vi "Exercise 2.2 DS18b20.vi"() -> ()   [LabVIEW 2014]
panel:
  out "Delay ms":u32
  out "C Chart":dbl(graph)=34.187
  out "C Meter":dbl(knob)=34.187 scale=15.0..40.0
  in  "error in (no error)":errorcluster
  out "error out":errorcluster
  out "Active":bool
  out "c":dbl=34.187
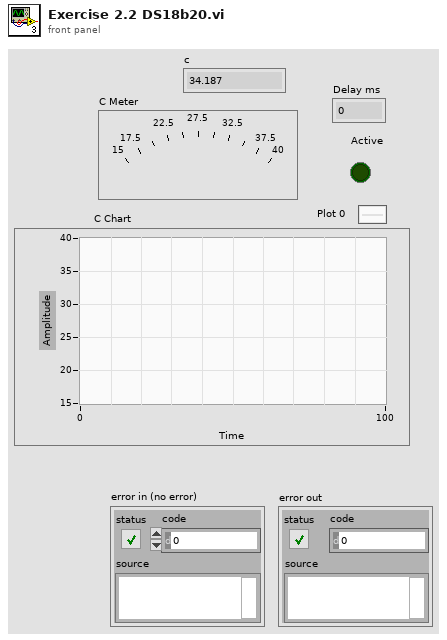
[diagram p1: front panel]
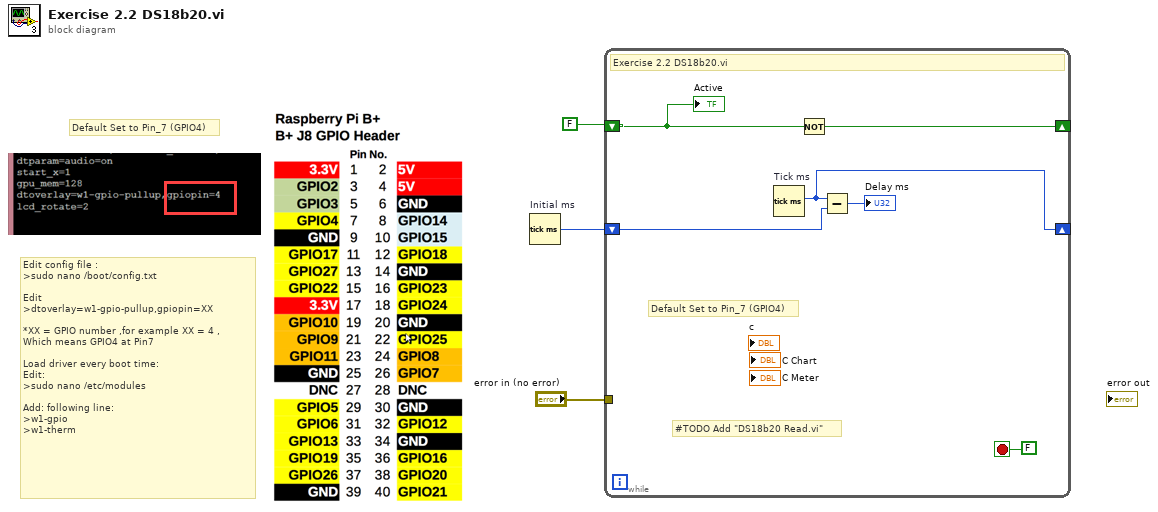
[diagram p0: block diagram]
diagram:
  # "Default Set to Pin_7 (GPIO4)"
  # "Edit config file :\n>sudo nano /boot/config.txt\n\nEdit\n>dtoverlay=w1-gpio-pullup,gpiopin=XX\n\n*XX = GPIO number ,for example XX = 4 ,\nWhich means GPIO4 at Pin7\n\nLoad driver every boot time:\nEdit:\n>sudo nano /etc/modules \n\nAdd: following line: \n>w1-gpio\n>w1-therm"
  n1 = Tick Count (ms) "Initial ms"() -> (millisecond timer value=w1:u32)
  n2 = while {
    tunnel: "error in (no error)" -> [_]
    shift-right: [w8] -> _
    shift-left: FALSE -> [w7]
    shift-right: [w5] -> _
    shift-left: w1 -> [w6]
    stop <- FALSE stop-if-true
    # "#TODO Add \"DS18b20 Read.vi\""
    # "Default Set to Pin_7 (GPIO4)"
    # "Exercise 2.2 DS18b20.vi"
    n3 = Tick Count (ms) "Tick ms"() -> (millisecond timer value=w5:u32)
    n4 = Not(x=w7) -> (.not. x?=w8:bool)
    n5 = Subtract(x=w5, y=w6) -> (x-y=→"Delay ms":u32)
    "Active" <- w7
  }
